vi "Signal Processing - Above Threshold.vi"(10 "Threshold":dbl, 11 "signal in":waveform(dbl)) -> (3 "Output":i32)   [LabVIEW 2010, in "Core SubVIs.lvlib"]
uses:
  Core SubVIs.lvlib
  <vilib>/Waveform/WDTOps.llb/WDT Waveform to XY Pairs DBL.vi
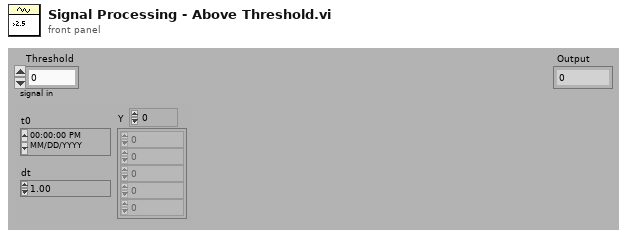
[diagram p1: front panel]
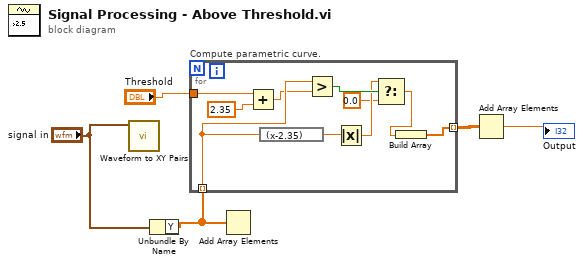
[diagram p0: block diagram]
diagram:
  n1 = call-poly <vilib>:"Waveform to XY Pairs.vi"("waveform in"="signal in") -> ()  [unwired: 8 in, 3 out]
  n2 = Unbundle By Name("signal in") -> ("Y"=w3:dbl[])
  n3 = for "Compute parametric curve." {
    tunnel: [w15] -> w5 mode=indexing
    tunnel: w3 -> [w12] mode=indexing
    tunnel: "Threshold" -> [w13]
    n4 = Add(x=w13, y=2.35) -> (x+y=w11:dbl)
    n5 = expression code="(x-2.35)"(w12) -> (w10:dbl)
    n6 = Greater?(x=w12, y=w11) -> (0:w9:bool)
    n7 = Absolute Value(x=w10) -> (abs(x)=w8:dbl)
    n8 = Select(t=w8, s=w9, f=0.0) -> (s? t:f=w6:dbl)
    n9 = Build Array(w6) -> (w15:dbl[])
  }
  n10 = Add Array Elements(numeric array=w3) -> ()  [unwired: 1 out]
  n11 = Add Array Elements(numeric array=w5) -> (sum=→"Output":dbl)
